vi "UDCReadSetting.vi"(7 "valueLen":i32, 8 "Error In":errorcluster, 9 "value":string, 10 "name":string, 11 "clientID":string) -> (0 "Error Out":errorcluster, 3 "Value Length":i32)   [LabVIEW 2017, in "niceiplib.lvlib"]
doc: "This API is used to read the setting either from registry or from the server. \n\nThe parameters are \n\n clientId Id of the client. Use the @p clientId of UDCStart(). Passing @p NULL will fetch the global settings.\n name Name of the setting.\n value Pass the pre-allocated @p char buffer to get the value (as string) back. Pass this as NULL pointer, then the length will be returned as part of the API.\n valueLen Maximum size of the value buffer. Not applicable, if the @param value is @p NULL.\n Returns Length of the value string in bytes."
uses:
  <vilib>/UDC/niceiplib.lvlib
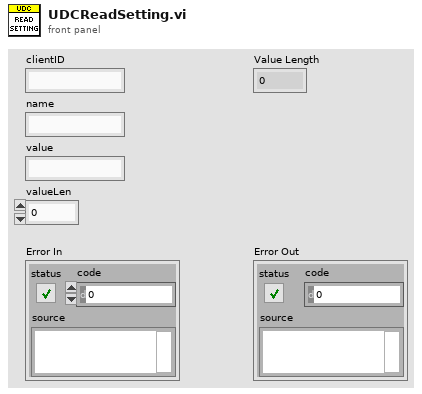
[diagram p1: front panel]
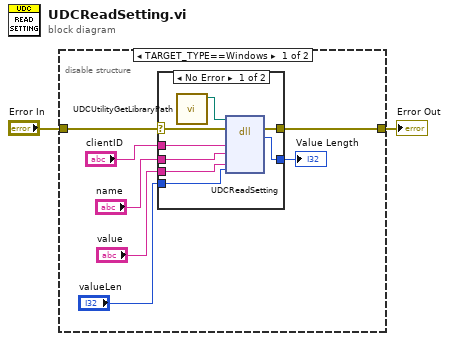
[diagram p0: block diagram]
diagram:
  n1 = disable-structure shown="TARGET_TYPE==Windows" {
    disable-tunnel: [w6 w19] -> w2
    disable-tunnel: "Error In" -> [w4 w19]
    frame condition #0 (active) {
      n2 = case shown="No Error" w4 {
        selector: w4 -> [w12 w18]
        tunnel: "clientID" -> [w17 _]
        tunnel: "name" -> [w16 _]
        tunnel: "valueLen" -> [w15 _]
        tunnel: [w14 w18] -> w6
        tunnel: "value" -> [w13 _]
        tunnel: [w11 _] -> w3
        frame No Error {
          n3 = call <vilib>:"UDCUtilityGetLibraryPath.vi"() -> ("Library Path"=w10:path)  [unwired: 11 in]
          n4 = dll-call lib="C:/2013LabVIEWCode/dist/vi.lib/UDC/niceiplib.*" fn="UDCReadSetting"(path in=w10, error in=w12, "clientID"=w17, "name"=w16, "value"=w13, "valueLen"=w15) -> (error out=w14:errorcluster, "Value Length"=w11:i32)  [unwired: 5 in, 1 out]
        }
        frame Error {
        }
      }
      "Value Length" <- w3
    }
    frame condition #1 {
    }
  }
  "Error Out" <- w2
